vi "EndOfMove-2.vi"(0 "InProgressIN":string[](array[string]), 2 "String in":string) -> (7 "InProgressOUT":string[](array[string]), 10 "InProgress":bool)   [LabVIEW 2013]
uses:
  <vilib>/regexp/Match Regular Expression.xnode
panel:
  out "Del":bool
  out "compare":bool
  out "add":bool
  in  "number":string
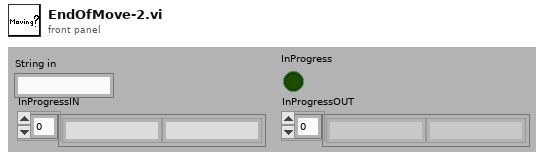
[diagram p1: front panel]
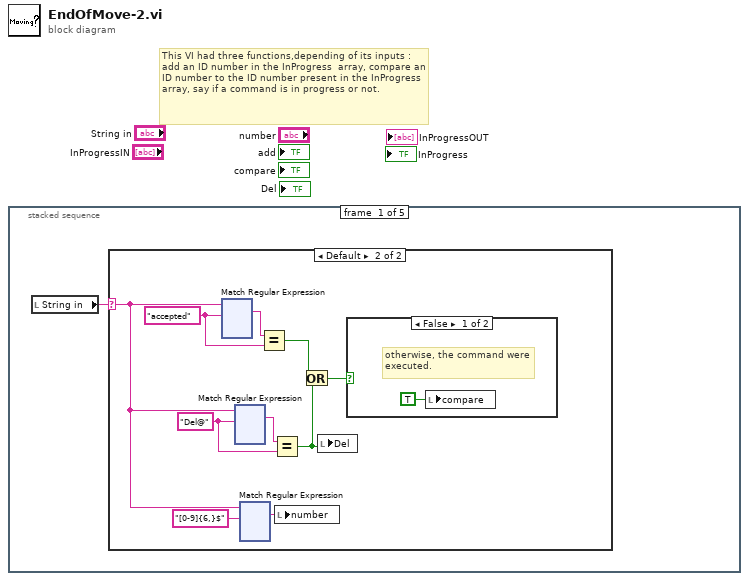
[diagram p0: block diagram]
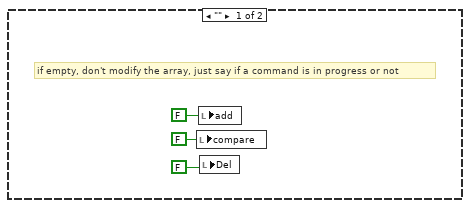
[diagram p2: hidden frame]
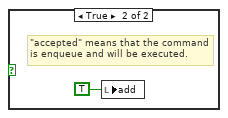
[diagram p3: hidden frame]
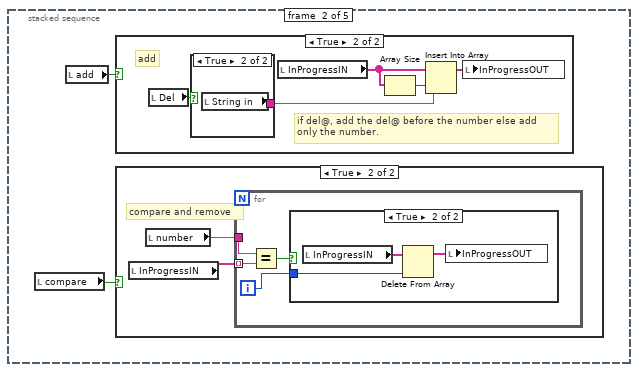
[diagram p4: hidden frame]
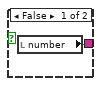
[diagram p8: hidden frame]
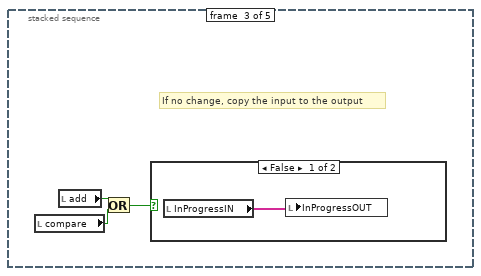
[diagram p9: hidden frame]
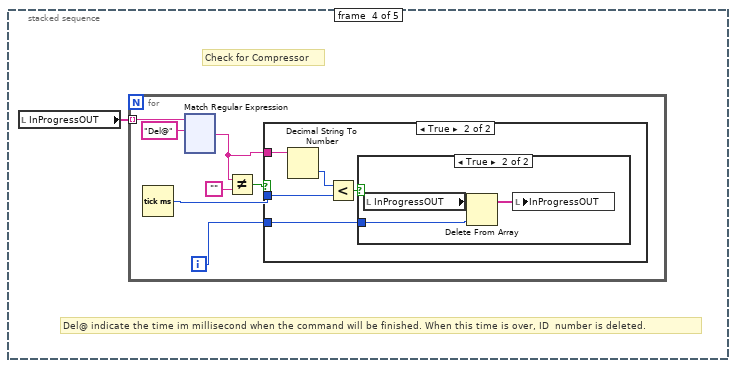
[diagram p11: hidden frame]
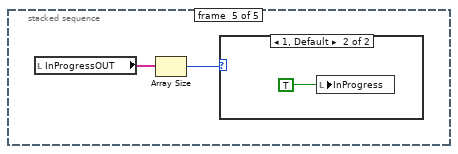
[diagram p14: hidden frame]
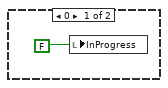
[diagram p15: hidden frame]
diagram:
  # "This VI had three functions,depending of its inputs : add an ID number in the InProgress  array, compare an ID number to the ID number present in the InProgress array, say if a command is in progress or not."
  n1 = stacked-sequence {
    frame #0 {
      n2 = local read "String in"() -> (w1:string)
      n3 = case shown="Default" w1 {
        selector: w1 -> [_ w8]
        frame "" {
          # "if empty, don't modify the array, just say if a command is in progress or not"
          n4 = local write "compare"(FALSE ("compare")) -> ()
          n5 = local write "add"(FALSE ("add")) -> ()
          n6 = local write "Del"(FALSE ("compare")) -> ()
        }
        frame Default {
          w9 = "Del@" ("regular expression")
          w13 = "accepted" ("regular expression")
          n7 = xnode "Match Regular Expression"("input string"=w8, "regular expression"=w13) -> ("whole match"=w14:string)  [unwired: 2 in, 6 out]
          n8 = xnode "Match Regular Expression"("input string"=w8, "regular expression"=w9) -> ("whole match"=w10:string)  [unwired: 2 in, 6 out]
          n9 = xnode "Match Regular Expression"("input string"=w8, "regular expression"="[0-9]{6,}$") -> ("whole match"=w11:string)  [unwired: 2 in, 6 out]
          n10 = Equal?(x=w14, y=w13) -> (x = y?=w7:bool)
          n11 = Equal?(x=w10, y=w9) -> (x = y?=w5:bool)
          n12 = local write "number"(w11) -> ()
          n13 = Or(x=w7, y=w5) -> (x .or. y?=w6:bool)
          n14 = local write "Del"(w5) -> ()
          n15 = case shown="False" w6 {
            frame False {
              # "otherwise, the command were executed."
              n16 = local write "compare"(TRUE ("compare")) -> ()
            }
            frame True {
              # "\"accepted\" means that the command is enqueue and will be executed."
              n17 = local write "add"(TRUE ("add")) -> ()
            }
          }
        }
      }
    }
    frame #1 {
      n18 = local read "compare"() -> (w350:bool)
      n19 = local read "add"() -> (w351:bool)
      n20 = case shown="True" w351 {
        frame False {
        }
        frame True {
          # "if del@, add the del@ before the number else add only the number."
          # "add"
          n21 = local read "Del"() -> (w362:bool)
          n22 = case shown="True" w362 {
            tunnel: [w366 w367] -> w361
            frame False {
              n23 = local read "number"() -> (w366:string)
            }
            frame True {
              n24 = local read "String in"() -> (w367:string)
            }
          }
          n25 = local read "InProgressIN"() -> (w364:string[])
          n26 = Array Size(array=w364) -> (size(s)=w365:i32)
          n27 = Insert Into Array(array=w364, index=w365, new element=w361) -> (w363:string[])
          n28 = local write "InProgressOUT"(w363) -> ()
        }
      }
      n29 = case shown="True" w350 {
        frame False {
        }
        frame True {
          # "compare and remove"
          n30 = local read "InProgressIN"() -> (w353:string[])
          n31 = local read "number"() -> (w352:string)
          n32 = for {
            tunnel: w353 -> [w356] mode=indexing
            tunnel: w352 -> [w354]
            i -> [w355]
            n33 = Equal?(x=w354, y=w356) -> (x = y?=w357:bool)
            n34 = case shown="True" w357 {
              tunnel: w355 -> [_ w358]
              frame False {
              }
              frame True {
                n35 = local read "InProgressIN"() -> (w360:string[])
                n36 = Delete From Array(array=w360, index=w358) -> (array with subset deleted=w359:string[])  [unwired: 1 in, 1 out]
                n37 = local write "InProgressOUT"(w359) -> ()
              }
            }
          }
        }
      }
    }
    frame #2 {
      # "If no change, copy the input to the output"
      n38 = local read "compare"() -> (w368:bool)
      n39 = local read "add"() -> (w369:bool)
      n40 = Or(x=w369, y=w368) -> (x .or. y?=w370:bool)
      n41 = case shown="False" w370 {
        frame False {
          n42 = local read "InProgressIN"() -> (w371:string[])
          n43 = local write "InProgressOUT"(w371) -> ()
        }
        frame True {
        }
      }
    }
    frame #3 {
      # "Del@ indicate the time im millisecond when the command will be finished. When this time is over, ID  number is deleted."
      # "Check for Compressor"
      n44 = local read "InProgressOUT"() -> (w372:string[])
      n45 = for {
        tunnel: w372 -> [w379] mode=indexing
        i -> [w374]
        n46 = Tick Count (ms)() -> (millisecond timer value=w375:u32)
        n47 = xnode "Match Regular Expression"("input string"=w379, "regular expression"="Del@") -> ("after match"=w376:string)  [unwired: 2 in, 6 out]
        n48 = Not Equal?(x=w376, y="") -> (x != y?=w373:bool)
        n49 = case shown="True" w373 {
          tunnel: w376 -> [_ w384]
          tunnel: w375 -> [_ w382]
          tunnel: w374 -> [_ w380]
          frame False {
          }
          frame True {
            n50 = Decimal String To Number(string=w384) -> (number=w383:i32)  [unwired: 3 out]
            n51 = Less?(x=w383, y=w382) -> (x < y?=w381:bool)
            n52 = case shown="True" w381 {
              tunnel: w380 -> [_ w386]
              frame False {
              }
              frame True {
                n53 = local read "InProgressOUT"() -> (w387:string[])
                n54 = Delete From Array(array=w387, index=w386) -> (array with subset deleted=w385:string[])  [unwired: 1 in, 1 out]
                n55 = local write "InProgressOUT"(w385) -> ()
              }
            }
          }
        }
      }
    }
    frame #4 {
      n56 = local read "InProgressOUT"() -> (w500:string[])
      n57 = Array Size(array=w500) -> (size(s)=w499:i32)
      n58 = case shown="1, Default" w499 {
        frame 0 {
          n59 = local write "InProgress"(FALSE) -> ()
        }
        frame 1, Default {
          n60 = local write "InProgress"(TRUE) -> ()
        }
      }
    }
  }
